vi "get Userinfo List.vi"(2 "userinfo list":T1, 8 "error in (no error)":errorcluster, 11 "[User] Userinfo in":refnum<class "[User] Userinfo.lvclass">) -> (0 "error out":errorcluster, 3 "[User] Userinfo out":refnum<class "[User] Userinfo.lvclass">)   [LabVIEW 2020, in "[User] Userinfo.lvclass"]
uses:
  [User] Userinfo.lvclass
  Control/userinfo list.ctl
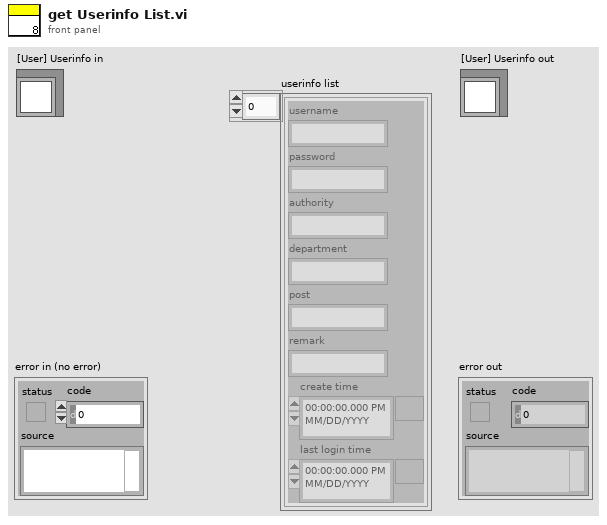
[diagram p1: front panel]
types:
  T1 = typedef "[User] Userinfo.lvclass/userinfo list.ctl" = cluster{"username":string, "password":string, "authority":string, "department":string, "post":string, "remark":string, "create time":timestamp, "last login time":timestamp}[]
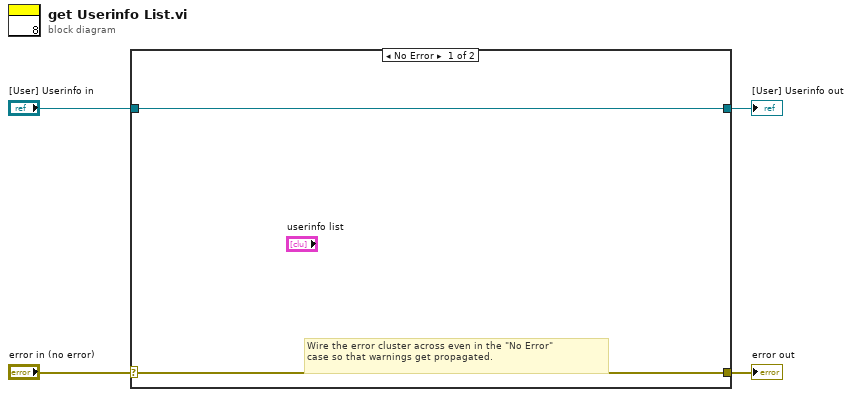
[diagram p0: block diagram]
diagram:
  n1 = case shown="No Error" "error in (no error)" {
    selector: "error in (no error)" -> [w5 w8]
    tunnel: [w5 w8] -> w3
    tunnel: [w6 w7] -> w1
    tunnel: "[User] Userinfo in" -> [w6 w7]
    frame No Error {
      # "Wire the error cluster across even in the \"No Error\"\ncase so that warnings get propagated."
    }
    frame Error {
    }
  }
  "error out" <- w3
  "[User] Userinfo out" <- w1
